vi "Destroy.vi"(0 "reference in":refnum<class "RemoteControl.lvclass">, 11 "Error In":errorcluster) -> (4 "reference out":refnum<class "RemoteControl.lvclass">, 15 "Error Out":errorcluster)   [LabVIEW 2024, in "RemoteControl.lvclass"]
uses:
  RemoteControl.lvclass/RemoteControl.ctl
  RemoteControl.lvclass
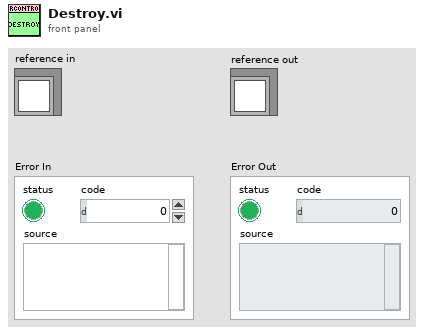
[diagram p1: front panel]
types:
  T1 = typedef "G4BaseTemplate_Simple_5x6x5.lvclass/ObjectAttributes.ctl" = cluster{"Attribute1":dbl}
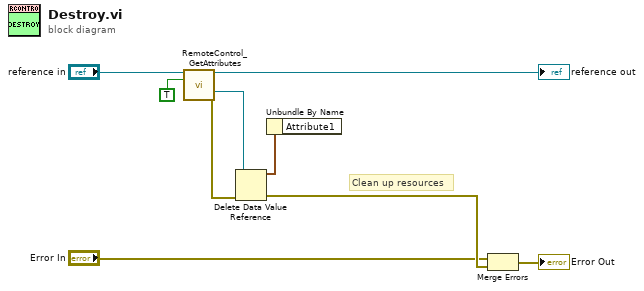
[diagram p0: block diagram]
diagram:
  # "Clean up resources"
  n1 = call "RemoteControl_GetAttributes.vi"("reference in"="reference in", "OnlyGetDvrReference(False)"=TRUE) -> ("reference out"=→"reference out":refnum<class "RemoteControl.lvclass">, "DataRef"=w5:refnum<data-value>, "Error Out"=w6:errorcluster)  [unwired: 10 in, 1 out]
  n2 = Delete Data Value Reference(data value reference=w5, error in=w6) -> (data value=w1:T1, error out=w4:errorcluster)
  n3 = Unbundle By Name(w1) -> ()  [unwired: 1 out]
  n4 = Merge Errors("Error In", w4) -> (→"Error Out":errorcluster)
